vi "Test Errors Are Cleared.vi"(8 "error in (no error)":errorcluster, 11 "Test Case In":refnum<class "Error Handler Tests.lvclass">) -> (0 "error out":errorcluster, 3 "Test Case Out":refnum<class "Error Handler Tests.lvclass">)   [LabVIEW 2020, in "Error Handler Tests.lvclass"]
uses:
  Error Handler Tests.lvclass
  Error Handler Tests.lvclass/Error Handler Tests.ctl
  source/User Interface/Process/Process.lvclass
  <vilib>/Astemes/LUnit/Test Case.lvclass
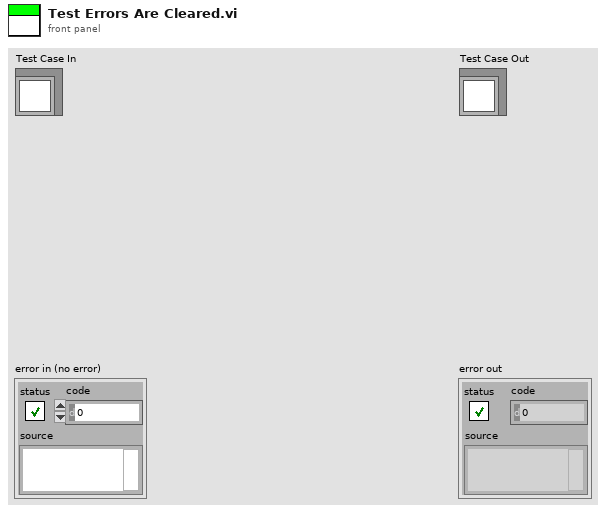
[diagram p1: front panel]
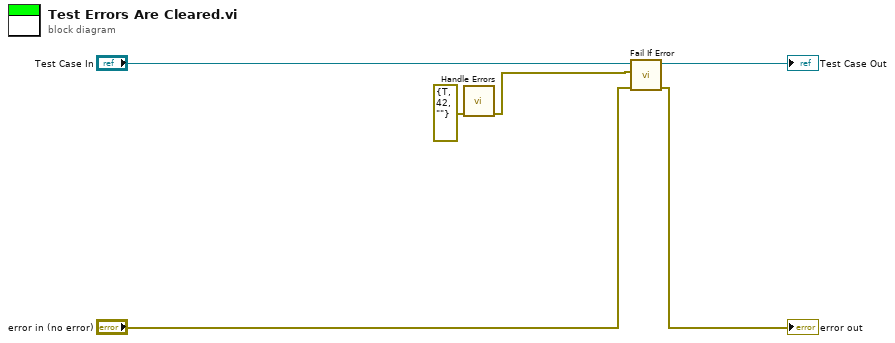
[diagram p0: block diagram]
diagram:
  n1 = call "Handle Errors.vi"("error in (no error)"=errorcluster {"status"=TRUE, "code"=42, "source"=""}) -> ("error out"=w2:errorcluster)  [unwired: 10 in]
  n2 = call <vilib>:"Fail If Error.vi"("error in (no error)"="error in (no error)", "Assert error"=w2, "LUnit Test Case In"="Test Case In") -> ("error out"=→"error out":errorcluster, "LUnit Test Case Out"=→"Test Case Out":refnum<class "Error Handler Tests.lvclass">)  [unwired: 7 in]
